vi "HEWH Terminate Draw Valve States.vi"(2 "Test Complete?":bool, 4 "Refnum in":T1, 5 "Station ID":T2=enum."A", 6 "Debug":bool, 7 "LV Program":T3=enum."HEWH", 8 "Error In":errorcluster, 9 "Stop Intellifaucet?":bool=TRUE, 10 "Pressurize Tank?":bool, 11 "MW100 In":refnum<visa-resource-name>="MW100") -> (0 "Error Out":errorcluster, 3 "MW100 Out":refnum<visa-resource-name>)   [LabVIEW 2016]
uses:
  Utility/Save File/File Setup (Public)/Type Definition/Save File DOE LabView Program.ctl
  Type Definitions/Station ID Selector.ctl
  Type Definitions/HEWH Normally Open Valve Control.ctl
  Type Definitions/HEWH Valve Bank Positions.ctl
  Utility/Save File/File Setup.lvlib
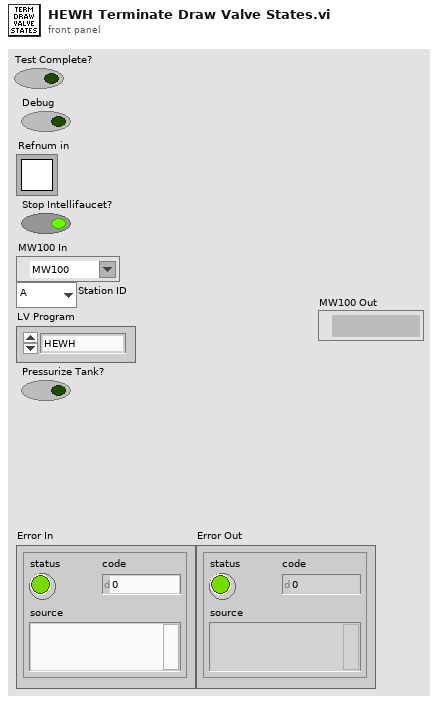
[diagram p1: front panel]
types:
  T1 = typedef "Semaphore RefNum" = refnum<k1>
  T2 = typedef "Station ID Selector.ctl" = enum16{"", "A", "B", "C", "D", "Global"}
  T3 = typedef "File Setup.lvlib/Save File DOE LabView Program.ctl" = enum16{"No Name Found", "DOE Stand", "Dishwasher Kitchen", "Portable Stand", "HEWH", "Dryer", "Dryer WILT", "HCC", "PRAT", "HEWH RLT", "Refrigeration"}
  T4 = typedef "HEWH Normally Open Valve Control.ctl" = string
  T5 = typedef "HEWH Valve Bank Positions.ctl" = enum16{"Heating", "Purge", "Resting", "Draw"}
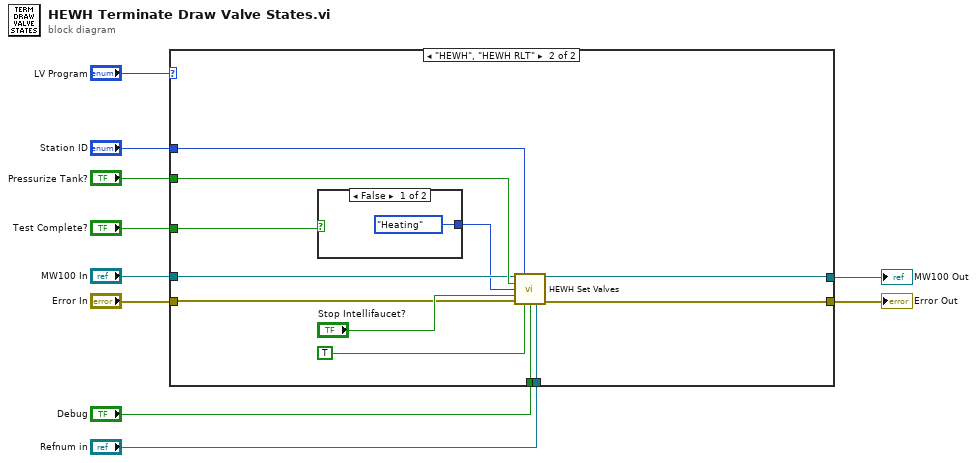
[diagram p0: block diagram]
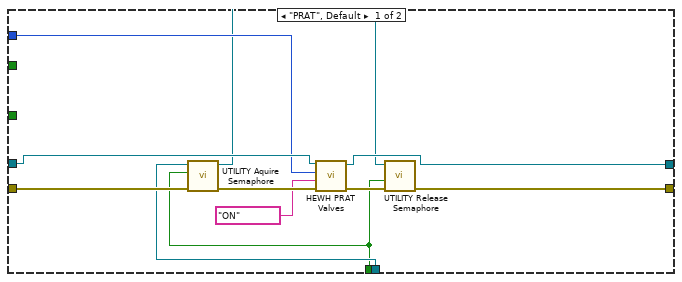
[diagram p2: hidden frame]
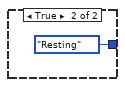
[diagram p3: hidden frame]
diagram:
  n1 = case shown="\"HEWH\", \"HEWH RLT\"" "LV Program" {
    tunnel: "Pressurize Tank?" -> [_ w33]
    tunnel: "Error In" -> [w18 w31]
    tunnel: [w15 w24] -> w9
    tunnel: "MW100 In" -> [w21 w30]
    tunnel: "Station ID" -> [w20 w29]
    tunnel: [w19 w23] -> w5
    tunnel: "Debug" -> [w12 w26]
    tunnel: "Refnum in" -> [w13 w25]
    tunnel: "Test Complete?" -> [_ w22]
    frame "PRAT", Default {
      n2 = call "UTILITY Aquire Semaphore.vi"("error in (no error)"=w18, "Debug"=w12, "Refnum in"=w13) -> ("error out"=w17:errorcluster, "Refnum out"=w14:T1)  [unwired: 6 in, 1 out]
      n3 = call "HEWH PRAT Valves.vi"("error in (no error)"=w17, "Normally Open Valve"=T4 "ON", "Station ID"=w20, "MW100 In"=w21) -> ("error out"=w16:errorcluster, "MW100 Out"=w19:refnum<visa-resource-name>)  [unwired: 6 in]
      n4 = call "UTILITY Release Semaphore.vi"("error in (no error)"=w16, "Debug"=w12, "Refnum in"=w14) -> ("error out"=w15:errorcluster)  [unwired: 8 in]
    }
    frame "HEWH", "HEWH RLT" {
      n5 = case shown="False" w22 {
        tunnel: [HEWH_Valve_Bank_Positions."Heating" ("Valve Bank Setting") HEWH_Valve_Bank_Positions."Resting" ("Valve Bank Setting")] -> w28
        frame False {
        }
        frame True {
        }
      }
      n6 = call "HEWH Set Valves.vi"("VISA session"=w30, "Station ID"=w29, "Pressurize Tank?"=w33, "Valve Bank Setting"=w28, "Stop Intellifaucet?"="Stop Intellifaucet?", "Error In"=w31, "Start Intellifaucet?"=TRUE, "Debug"=w26, "Refnum in"=w25) -> ("dup VISA session"=w23:refnum<visa-resource-name>, "Error Out"=w24:errorcluster)  [unwired: 5 in]
    }
  }
  "Error Out" <- w9
  "MW100 Out" <- w5
